vi "Memory.Pointer.Count to Size.Power of 2.vi"(7 "power of 2":i16, 11 "count":u64 format="%0d") -> (3 "size":u64 format="%08x bytes")   [LabVIEW 2016, in "Memory.lvlib" / "Memory.Pointer.lvclass"]
doc: "Upshifts <b>count</b> by the specified <b>power of 2</b> to get the size in bytes."
uses:
  Memory.Pointer.lvclass
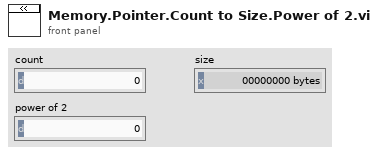
[diagram p1: front panel]
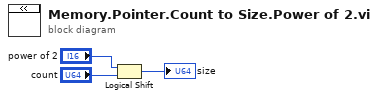
[diagram p0: block diagram]
diagram:
  n1 = Logical Shift(y="power of 2", x="count") -> (x << y=→"size":u64)
